vi "Configure Lamp.vi"(0 "VISA Resource Name":refnum<visa-resource-name>, 1 "Lamp Intensity (1.0 V)":dbl=1.0 format="%.3f", 5 "Device Number (1)":i32=1, 7 "Lamp Enabled (True)":bool=TRUE, 9 "Lamp Type (0: Transmitted)":enum16{"Transmitted", "Reflected"}(ring), 11 "error in (no error)":errorcluster {"code" format="%.0x"}) -> (4 "VISA Resource Name Out":refnum<visa-resource-name>, 15 "error out":errorcluster {"code" format="%.0x"})   [LabVIEW 2020, in "Olympus IX BX Series.lvlib"]
doc: "This VI configure lamp behaviors."
uses:
  Olympus IX BX Series.lvlib
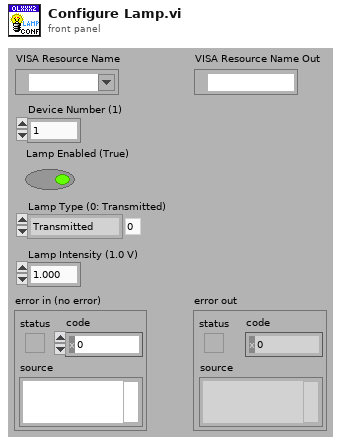
[diagram p1: front panel]
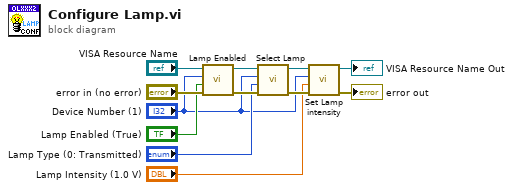
[diagram p0: block diagram]
diagram:
  n1 = call "Lamp Enabled.vi"("error in (no error)"="error in (no error)", "Lamp Enabled (True)"="Lamp Enabled (True)", "Device Number (1)"="Device Number (1)", "VISA Resource Name"="VISA Resource Name") -> ("error out"=w9:errorcluster, "VISA Resource Name Out"=w8:refnum<visa-resource-name>)  [unwired: 6 in]
  n2 = call "Select Lamp.vi"("error in (no error)"=w9, "Lamp Type (0: Transmitted)"="Lamp Type (0: Transmitted)", "Device Number (1)"="Device Number (1)", "VISA Resource Name"=w8) -> ("error out"=w6:errorcluster, "VISA Resource Name Out"=w5:refnum<visa-resource-name>)  [unwired: 6 in]
  n3 = call "Set Lamp intensity.vi"("error in (no error)"=w6, "Lamp Intensity (1.0 V)"="Lamp Intensity (1.0 V)", "Device Number (1)"="Device Number (1)", "VISA Resource Name"=w5) -> ("error out"=→"error out":errorcluster, "VISA Resource Name Out"=→"VISA Resource Name Out":refnum<visa-resource-name>)  [unwired: 6 in]
